vi "test_harness.vi"() -> ()   [LabVIEW 2019]
uses:
  Module/AI_Module_Data.ctl
  Module/Module_Data.ctl
  Module/DO_Module_Data.ctl
  USB-87Pn.lvclass
panel:
  out "Waveform Chart":T1(graph)
  in  "stop":bool
  out "AI float":sgl[][](array[numeric])
  in  "error in (no error)":errorcluster
  out "error out":errorcluster
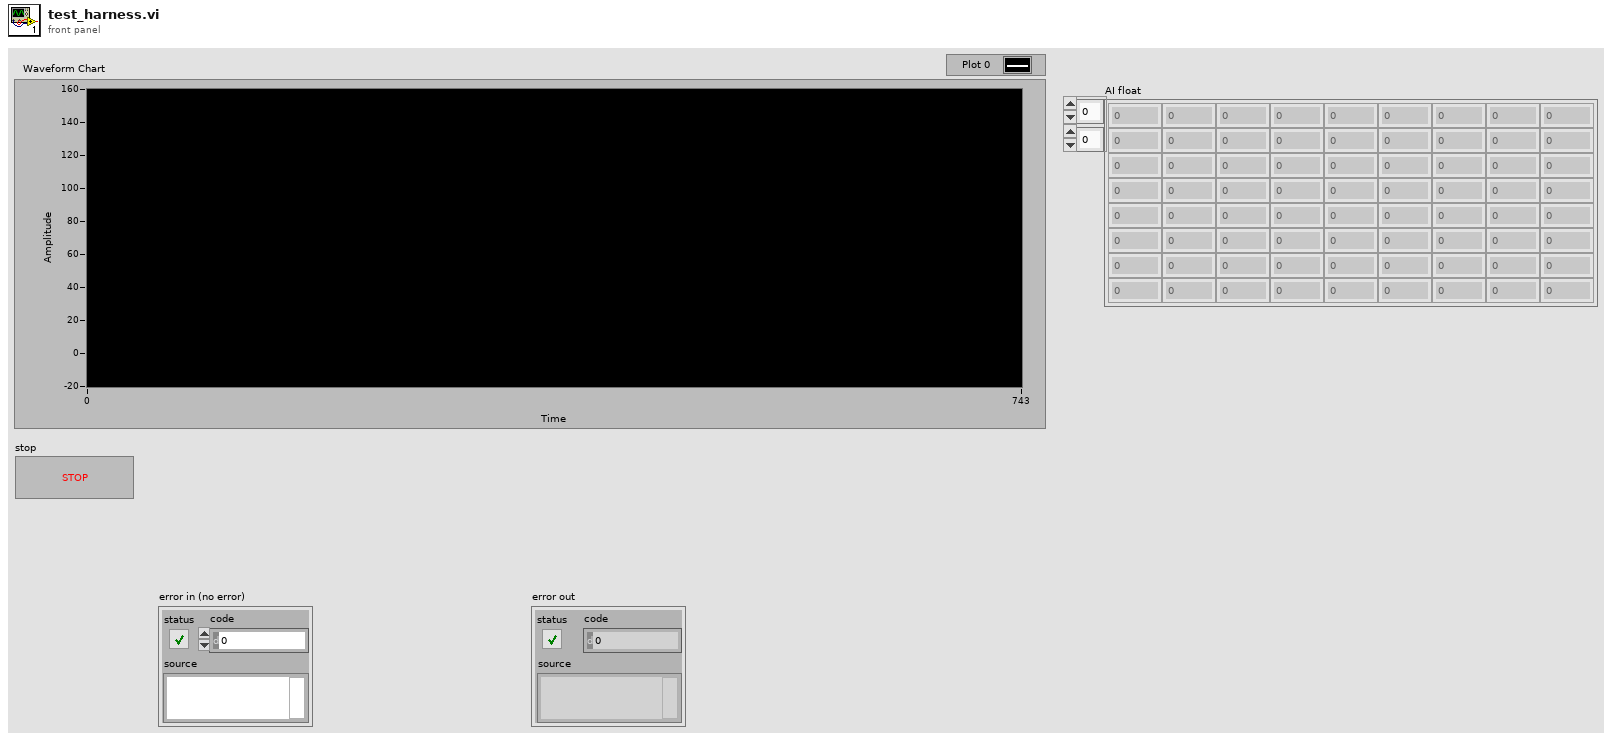
[diagram p1: front panel]
types:
  T1 = cluster{"[0]":sgl, "[1]":sgl, "[2]":sgl, "[3]":sgl, "[4]":sgl, "[5]":sgl, "[6]":sgl, "[7]":sgl, "[8]":sgl, "[9]":sgl, "[10]":sgl, "[11]":sgl, "[12]":sgl, "[13]":sgl, "[14]":sgl, "[15]":sgl, "[16]":sgl, "[17]":sgl, "[18]":sgl, "[19]":sgl, "[20]":sgl, "[21]":sgl, "[22]":sgl, "[23]":sgl, "[24]":sgl, "[25]":sgl, "[26]":sgl, "[27]":sgl, "[28]":sgl, "[29]":sgl, "[30]":sgl, "[31]":sgl}
  T2 = typedef "USB-87Pn.lvlib/USB-87Pn.lvclass/DO_Module_Data.ctl" = cluster{"Module_Data":T3, "DO_Channels":cluster{"Enabled":bool, "Alias":string}[]}
  T3 = typedef "USB-87Pn.lvlib/USB-87Pn.lvclass/Module_Data.ctl" = cluster{"Number of Channels":u8, "Address":i16, "Alias":string}
  T4 = typedef "USB-87Pn.lvlib/USB-87Pn.lvclass/AI_Module_Data.ctl" = cluster{"Module_Data":T3, "AI_Channels":cluster{"Enabled":bool, "Alias":string}[]}
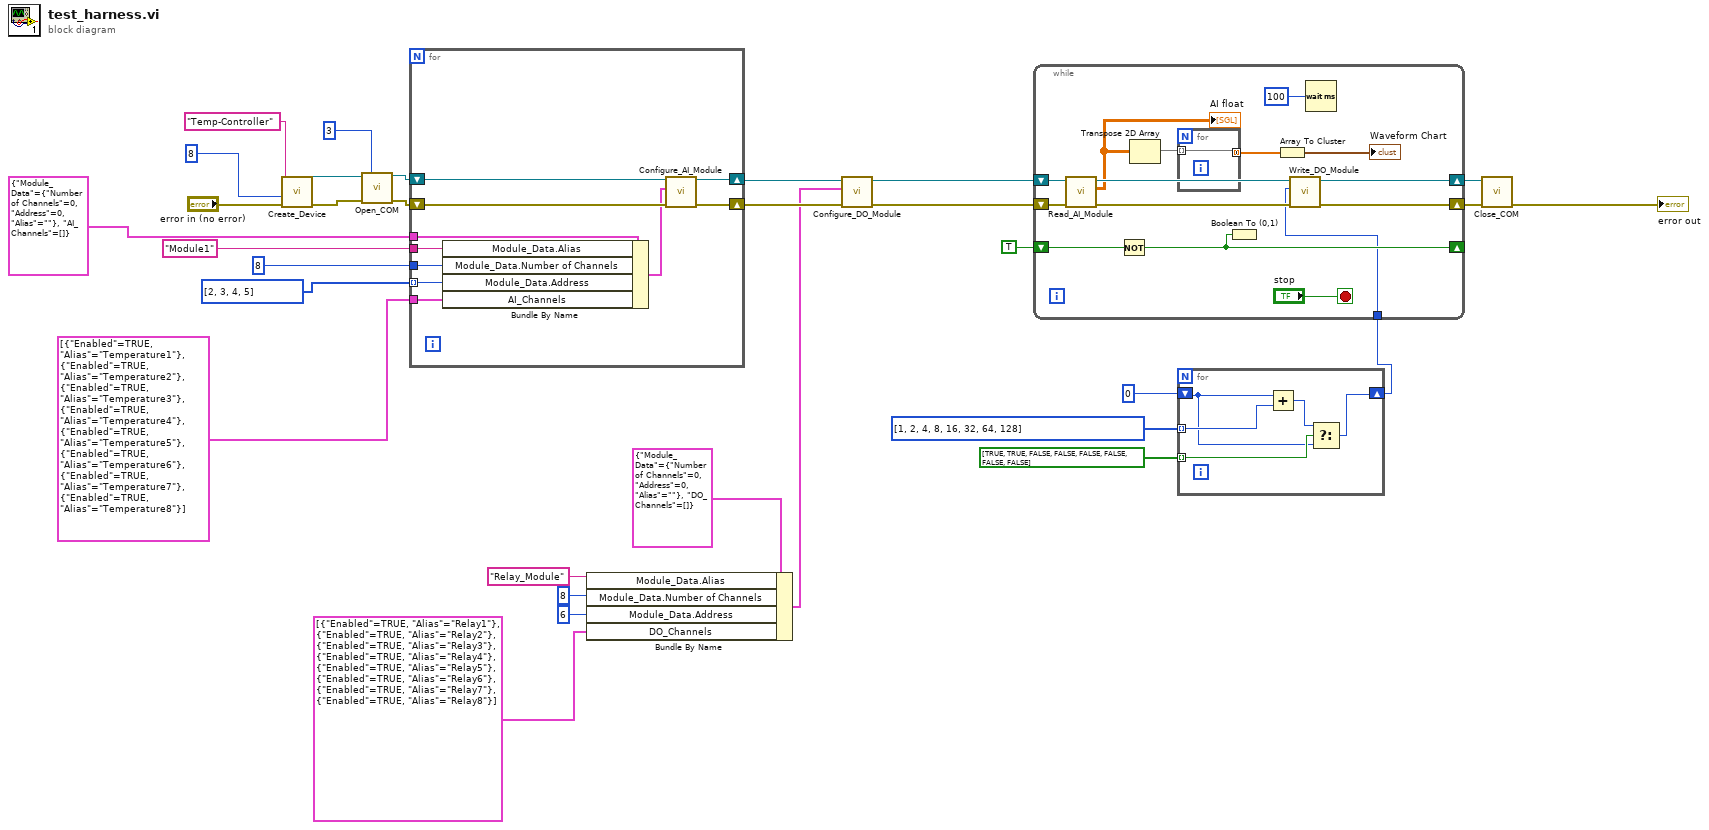
[diagram p0: block diagram]
diagram:
  n1 = call "Create_Device.vi"("error in (no error)"="error in (no error)", "Number of Slots"=i8 8, "Device Name"="Temp-Controller") -> ("error out"=w30:errorcluster, "87Pn out"=w31:refnum<class "USB-87Pn.lvclass">)  [unwired: 7 in]
  n2 = call "Open_COM.vi"("USB-87Pn in"=w31, "port number"=u8 3, "error in (no error)"=w30) -> ("USB-87Pn out"=w21:refnum<class "USB-87Pn.lvclass">, "error out"=w22:errorcluster)  [unwired: 11 in]
  n3 = for {
    shift-right: [w39] -> w15
    shift-left: w21 -> [w40]
    shift-right: [w38] -> w14
    shift-left: w22 -> [w41]
    tunnel: T4 {"Module_Data"={"Number of Channels"=0, "Address"=0, "Alias"=""}, "AI_Channels"=[]} ("AI_Module_Data") -> [w37]
    tunnel: "Module1" ("Module_Data.Alias") -> [w36]
    tunnel: u8 8 ("Module_Data.Number of Channels") -> [w35]
    tunnel: cluster{"Enabled":bool, "Alias":string}[] [{"Enabled"=TRUE, "Alias"="Temperature1"}, {"Enabled"=TRUE, "Alias"="Temperature2"}, {"Enabled"=TRUE, "Alias"="Temperature3"}, {"Enabled"=TRUE, "Alias"="Temperature4"}, {"Enabled"=TRUE, "Alias"="Temperature5"}, {"Enabled"=TRUE, "Alias"="Temperature6"}, {"Enabled"=TRUE, "Alias"="Temperature7"}, {"Enabled"=TRUE, "Alias"="Temperature8"}] ("AI_Channels") -> [w34]
    tunnel: i16[] [2, 3, 4, 5] -> [w32] mode=indexing
    n4 = Bundle By Name(cluster=w37, "Module_Data.Alias"=w36, "Module_Data.Number of Channels"=w35, "Module_Data.Address"=w32, "AI_Channels"=w34) -> (w33:T4)
    n5 = call "Configure_AI_Module.vi"("error in (no error)"=w41, "AI_Module_Data"=w33, "USB-87Pn"=w40) -> ("error out"=w38:errorcluster, "USB-87Pn"=w39:refnum<class "USB-87Pn.lvclass">)  [unwired: 7 in]
  }
  n6 = Bundle By Name(cluster=T2 {"Module_Data"={"Number of Channels"=0, "Address"=0, "Alias"=""}, "DO_Channels"=[]} ("DO_Module_Data"), "Module_Data.Alias"="Relay_Module", "Module_Data.Number of Channels"=u8 8, "Module_Data.Address"=i16 6, "DO_Channels"=cluster{"Enabled":bool, "Alias":string}[] [{"Enabled"=TRUE, "Alias"="Relay1"}, {"Enabled"=TRUE, "Alias"="Relay2"}, {"Enabled"=TRUE, "Alias"="Relay3"}, {"Enabled"=TRUE, "Alias"="Relay4"}, {"Enabled"=TRUE, "Alias"="Relay5"}, {"Enabled"=TRUE, "Alias"="Relay6"}, {"Enabled"=TRUE, "Alias"="Relay7"}, {"Enabled"=TRUE, "Alias"="Relay8"}]) -> (w10:T2)
  n7 = call "Configure_DO_Module.vi"("error in (no error)"=w14, "DO_Module_Data"=w10, "USB-87Pn in"=w15) -> ("error out"=w12:errorcluster, "USB-87Pn out"=w13:refnum<class "USB-87Pn.lvclass">)  [unwired: 7 in]
  n8 = for {
    tunnel: bool[] [TRUE, TRUE, FALSE, FALSE, FALSE, FALSE, FALSE, FALSE] -> [w46] mode=indexing
    tunnel: i32[] [1, 2, 4, 8, 16, 32, 64, 128] -> [w45] mode=indexing
    shift-right: [w42] -> w1
    shift-left: 0 -> [w43]
    n9 = Add(x=w43, y=w45) -> (x+y=w44:i32)
    n10 = Select(t=w44, s=w46, f=w43) -> (s? t:f=w42:i32)
  }
  n11 = while {
    shift-right: [w55] -> w24
    shift-left: w12 -> [w61]
    shift-right: [w56] -> w25
    shift-left: w13 -> [w60]
    shift-right: [w52] -> _
    shift-left: TRUE -> [w54]
    tunnel: w1 -> [w47]
    stop <- "stop" stop-if-true
    n12 = call "Read_AI_Module.vi"("error in (no error)"=w61, "USB-87Pn in"=w60) -> ("error out"=w57:errorcluster, "AI float"=w50:sgl[][], "USB-87Pn out"=w58:refnum<class "USB-87Pn.lvclass">)  [unwired: 7 in]
    "AI float" <- w50
    n13 = Not(x=w54) -> (.not. x?=w52:bool)
    n14 = Transpose 2D Array(2D array=w50) -> (transposed array=w51:sgl[][])
    n15 = for {
      tunnel: w51 -> [w62] mode=indexing
      tunnel: [w62] -> w49 mode=concatenating
    }
    n16 = Boolean To (0,1)(Boolean=w52) -> ()  [unwired: 1 out]
    n17 = Array To Cluster(array=w49) -> (cluster=→"Waveform Chart":T1)
    n18 = call "Write_DO_Module.vi"("error in (no error)"=w57, "DO_Value"=w47, "USB-87Pn in"=w58) -> ("error out"=w55:errorcluster, "USB-87Pn out"=w56:refnum<class "USB-87Pn.lvclass">)  [unwired: 7 in]
    n19 = Wait (ms)(milliseconds to wait=u32 100) -> ()  [unwired: 1 out]
  }
  n20 = call "Close_COM.vi"("error in (no error)"=w24, "USB-87Pn in"=w25) -> ("error out"=→"error out":errorcluster)  [unwired: 8 in, 1 out]
